vi "Build Description String.vi"(8 "error in (no error)":errorcluster, 11 "Disabled Assertion in":refnum<class "Disabled Assertion.lvclass">) -> (0 "error out":errorcluster, 2 "Description":string, 3 "Disabled Assertion out":refnum<class "Disabled Assertion.lvclass">)   [LabVIEW 2020, in "MacroAssert.lvlib" / "Disabled Assertion.lvclass"]
doc: "Builds a string to describe what <B>Step</B> does."
uses:
  Disabled Assertion.lvclass
  C:/Users/User/Documents/LabVIEW Data/Projects/MacroAssert/source/Classes/Control Assertion/Control Assertion.lvclass
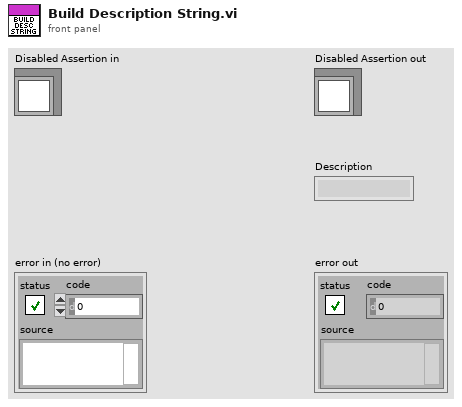
[diagram p1: front panel]
types:
  T1 = enum8{"Enabled", "Disabled", "Disabled and Grayed Out"}
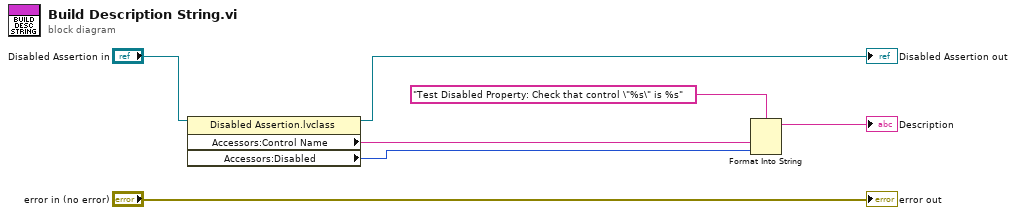
[diagram p0: block diagram]
diagram:
  n1 = property class="Disabled Assertion.lvclass"(reference="Disabled Assertion in") -> (reference out=→"Disabled Assertion out":refnum<class "Disabled Assertion.lvclass">, "Accessors:Control Name"=w5:string, "Accessors:Disabled"=w3:T1)  [unwired: 1 in, 1 out]
  n2 = Format Into String(format string="Test Disabled Property: Check that control \"%s\" is %s", w5, w3) -> (resulting string=→"Description":string)  [unwired: 2 in, 1 out]
  "error out" <- "error in (no error)"
